vi "triggerGlobalVarsWrite.vi"(0 "triggerTypes":T3, 1 "selectTrigger":T2, 2 "delay_10ns_ticks":u32, 3 "triggerEdge":T1=enum."true-false") -> ()   [LabVIEW 2014]
uses:
  Controls/triggerTypes.ctl
  Controls/selectTrigger.ctl
  Controls/triggerEdge.ctl
  <vilib>/rvi/Emulation/niFpgaSctlEmulationGetInTimedLoop.vi
  triggerGlobalVars.vi
  <vilib>/rvi/Emulation/niFpgaProcessEmulError.vi
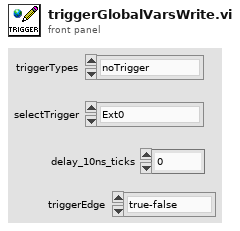
[diagram p1: front panel]
types:
  T1 = typedef "triggerEdge.ctl" = enum8{"either", "false-true", "true-false"}
  T2 = typedef "selectTrigger.ctl" = enum8{"Ext0", "Ext1", "Ext2", "Ext3", "Ext4", "Ext5", "Ext6", "Ext7", "Int0", "Int1", "Int2", "Int3", "Int4", "Int5", "Int6", "Int7"}
  T3 = typedef "triggerTypes.ctl" = enum16{"noTrigger", "singleHitDelay", "singleHit", "software", "sweep"}
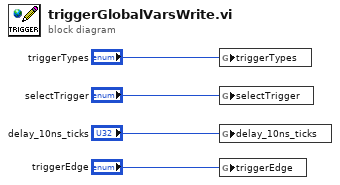
[diagram p0: block diagram]
diagram:
  n1 = global write "triggerGlobalVars.vi" "triggerTypes"("triggerTypes") -> ()
  n2 = global write "triggerGlobalVars.vi" "selectTrigger"("selectTrigger") -> ()
  n3 = global write "triggerGlobalVars.vi" "delay_10ns_ticks"("delay_10ns_ticks") -> ()
  n4 = global write "triggerGlobalVars.vi" "triggerEdge"("triggerEdge") -> ()
